vi "PauseResume.vi"(8 "error in":errorcluster, 11 "PauseResume Ref":refnum<vi>) -> (0 "error out":errorcluster, 3 "Data":string[][](array[string]))   [LabVIEW 2025, in "CAN-LIN Raw Bus Capture UI.lvlib"]
doc: "Get new data from the Table Buffer Queue, if the Plug-In is unpaused.\n\nDoes not wait for an element, only dequeues if elements are in the queue.\n\nIf the Update? is True then onyl checks the pause state. This means that if you want to ignore leftover packages when paused at shutdown, keep it on true."
uses:
  CAN-LIN Raw Bus Capture UI.lvlib
  Get Status.vi
  Dequeue Data.vi
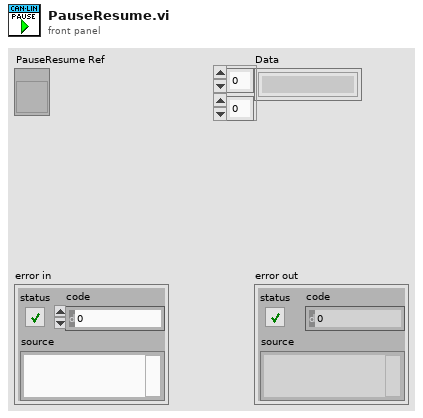
[diagram p1: front panel]
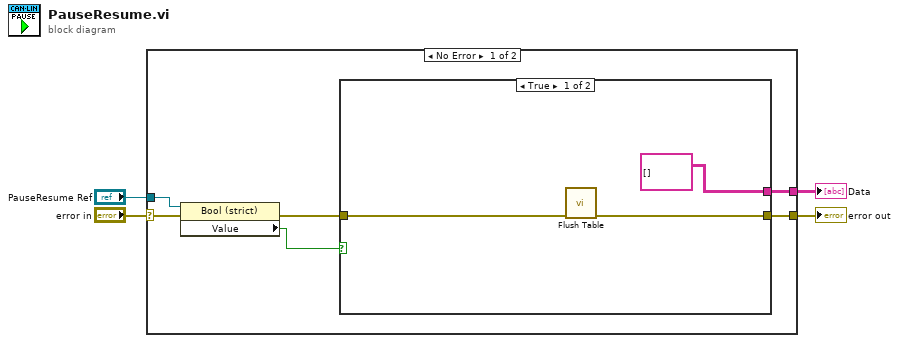
[diagram p0: block diagram]
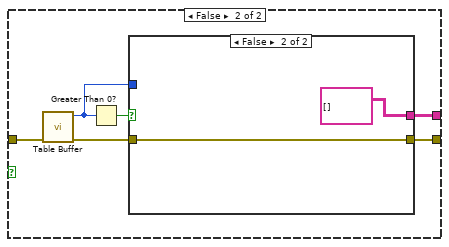
[diagram p2: hidden frame]
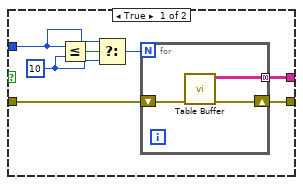
[diagram p3: hidden frame]
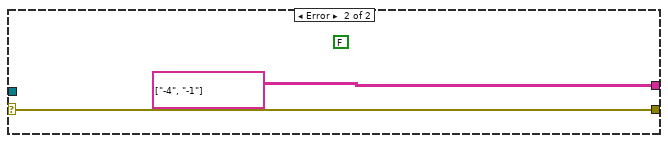
[diagram p4: hidden frame]
diagram:
  n1 = case shown="No Error" "error in" {
    selector: "error in" -> [w9 w33]
    tunnel: [w10 w33] -> w4
    tunnel: "PauseResume Ref" -> [w7 _]
    tunnel: [w6 string[][] [["-4", "-1"]] ("Data")] -> w1
    frame No Error {
      n2 = property class="Bool (strict)"(reference=w7, error in=w9) -> (error out=w8:errorcluster, "Value"=w5:bool)  [unwired: 1 out]
      n3 = case shown="True" w5 {
        tunnel: [w12 w19] -> w10
        tunnel: w8 -> [w11 w16]
        tunnel: [string[][] [] ("Data") w18] -> w6
        frame True {
          n4 = call "Flush Table.vi"("error in"=w11) -> ("error out"=w12:errorcluster)  [unwired: 10 in]
        }
        frame False {
          n5 = call-poly "Table Buffer.vi"("error in"=w16) -> ("error out"=w17:errorcluster, "Messages"=w14:i32)  [unwired: 9 in]
          n6 = Greater Than 0?(x=w14) -> (x > 0?=w15:bool)
          n7 = case shown="False" w15 {
            tunnel: [w26 w30] -> w19
            tunnel: w17 -> [w25 w30]
            tunnel: [w20 string[][] [] ("Data")] -> w18
            tunnel: w14 -> [w22 _]
            frame True {
              w23 = 10 ("y")
              n8 = Less Or Equal?(x=w22, y=w23) -> (x <= y?=w24:bool)
              n9 = Select(t=w22, s=w24, f=w23) -> (s? t:f=w21:i32)
              n10 = for {
                N: w21 -> [_]
                shift-right: [w29] -> w26
                shift-left: w25 -> [w28]
                tunnel: [w27] -> w20 mode=concatenating
                n11 = call-poly "Table Buffer.vi"("error in"=w28) -> ("error out"=w29:errorcluster, "Data"=w27:string[][])  [unwired: 9 in]
              }
            }
            frame False {
            }
          }
        }
      }
    }
    frame Error {
      (unwired) FALSE ("Value")
    }
  }
  "error out" <- w4
  "Data" <- w1
